vi "Get Deepest Path.vi"(8 "Error In":errorcluster, 11 "File Paths":path[](array[path])) -> (0 "Error Out":errorcluster, 1 "Path Tokens":i32, 2 "Deepest Path":path, 3 "Duplicate File Paths":path[](array[path]))   [LabVIEW 2014, in "LMH-Toolbox.lvlib"]
doc: "Given an array of file paths find the deepest path (ie the path containing the most path elements)."
uses:
  <vilib>/MakerHub/Toolbox/LMH-Toolbox.lvlib
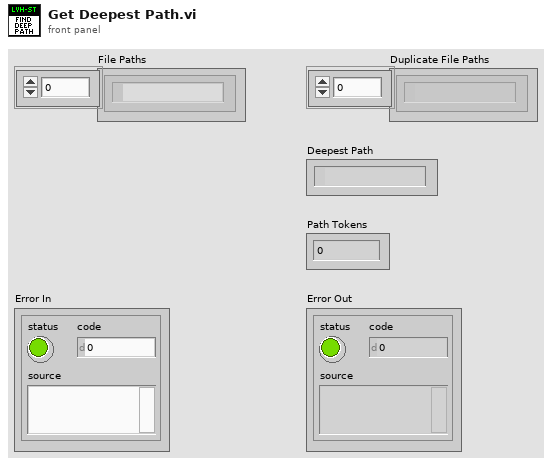
[diagram p1: front panel]
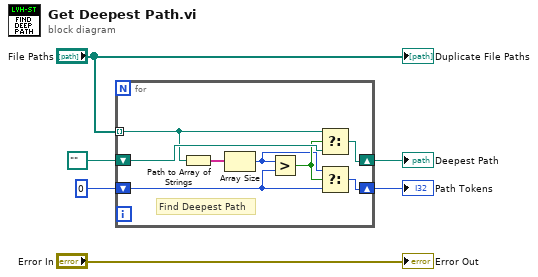
[diagram p0: block diagram]
diagram:
  n1 = for {
    tunnel: "File Paths" -> [w7] mode=indexing
    shift-right: [w13] -> w3
    shift-left: path "" -> [w14]
    shift-right: [w10] -> w5
    shift-left: 0 -> [w11]
    # "Find Deepest Path"
    n2 = Path to Array of Strings(0:w7) -> (2:w9:string[])  [unwired: 1 out]
    n3 = Array Size(array=w9) -> (size(s)=w8:i32)
    n4 = Greater?(x=w8, y=w11) -> (0:w12:bool)
    n5 = Select(t=w7, s=w12, f=w14) -> (s? t:f=w13:path)
    n6 = Select(t=w8, s=w12, f=w11) -> (s? t:f=w10:i32)
  }
  "Path Tokens" <- w5
  "Deepest Path" <- w3
  "Duplicate File Paths" <- "File Paths"
  "Error Out" <- "Error In"
